vi "Build Test File Paths.vi"(6 "Test Files":T1[](array[typedef]), 8 "Tests Folder Path":path, 9 "Runnable Test Selector":bool[](array[boolean]), 10 "Multiplier of runs":i32, 11 "Run All":bool) -> (3 "Test File Paths to Execute":path[](array[path]))   [LabVIEW 2018, in "Common Support.lvlib"]
uses:
  Common Support.lvlib
  Test File Path--cluster.ctl
panel:
  in  "All Test":bool
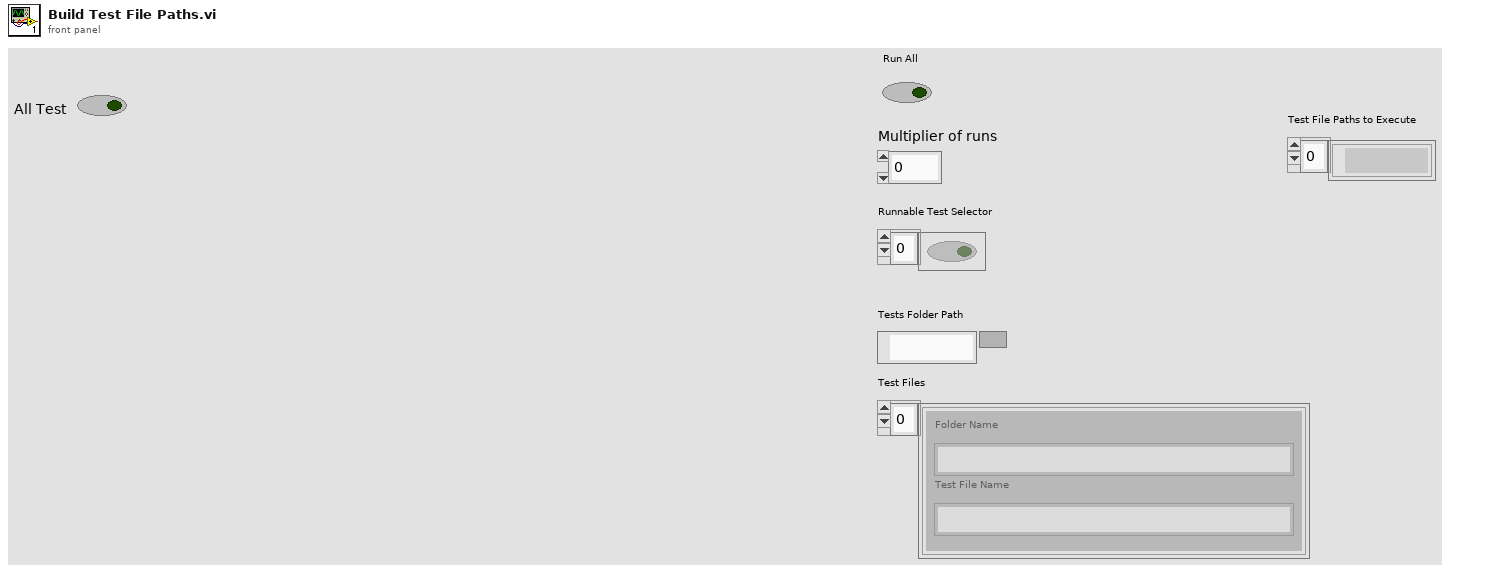
[diagram p1: front panel]
types:
  T1 = typedef "Common Support.lvlib/Test File Path--cluster.ctl" = cluster{"Folder Name":string, "Test File Name":string}
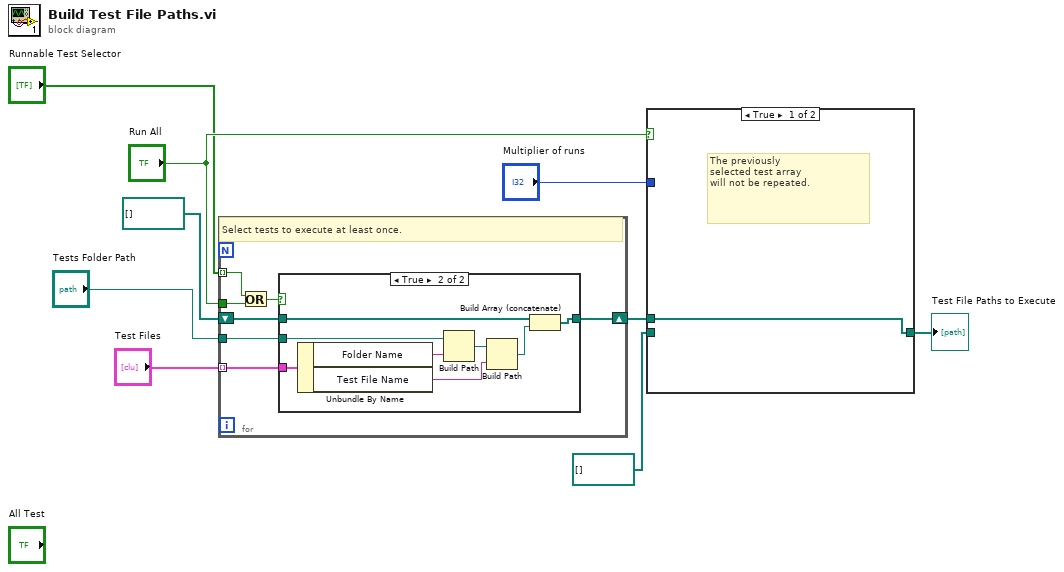
[diagram p0: block diagram]
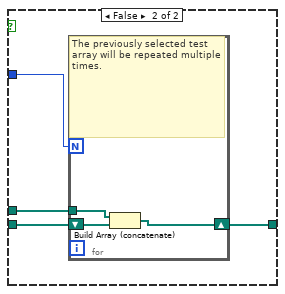
[diagram p2: hidden frame]
diagram:
  n1 = for {
    tunnel: "Test Files" -> [w16] mode=indexing
    tunnel: "Tests Folder Path" -> [w15]
    shift-right: [w13] -> w9
    shift-left: path[] [] -> [w14]
    tunnel: "Run All" -> [w12]
    tunnel: "Runnable Test Selector" -> [w10] mode=indexing
    # "Select tests to execute at least once."
    n2 = Or(x=w10, y=w12) -> (x .or. y?=w11:bool)
    n3 = case shown="True" w11 {
      tunnel: w16 -> [_ w25]
      tunnel: w15 -> [_ w22]
      tunnel: w14 -> [w17 w19]
      tunnel: [w17 w18] -> w13
      frame False {
      }
      frame True {
        n4 = Unbundle By Name(w25) -> ("Folder Name"=w24:string, "Test File Name"=w23:string)
        n5 = Build Path(base path=w22, name or relative path=w24) -> (appended path=w21:path)
        n6 = Build Path(base path=w21, name or relative path=w23) -> (appended path=w20:path)
        n7 = Build Array (concatenate)(w19, w20) -> (w18:path[])
      }
    }
  }
  n8 = case shown="True" "Run All" {
    tunnel: "Multiplier of runs" -> [_ w27]
    tunnel: w9 -> [w26 w30]
    tunnel: path[] [] -> [_ w29]
    tunnel: [w26 w28] -> w1
    frame True {
      # "The previously \nselected test array \nwill not be repeated."
    }
    frame False {
      n9 = for {
        N: w27 -> [_]
        tunnel: w30 -> [w32]
        shift-right: [w33] -> w28
        shift-left: w29 -> [w31]
        # "The previously selected test array will be repeated multiple times."
        n10 = Build Array (concatenate)(w32, w31) -> (w33:path[])
      }
    }
  }
  "Test File Paths to Execute" <- w1
